vi "parse_GPGSA.vi"(0 "NMEA GPGSA String":string) -> (1 "2D3D_Automatic?":bool, 2 "New Fix Quality":T1, 3 "Valid GPS Fix?":bool)   [LabVIEW 2010]
doc: "Pass this VI an NMEA sentence and it will parse it as if it's a GPGGA sentence.\nThe Valid GPS output will be false if there's no fix or if it's not a GPGGA sentence."
uses:
  _types/FixQuality.ctl
panel:
  out "$GPGGA Code":string
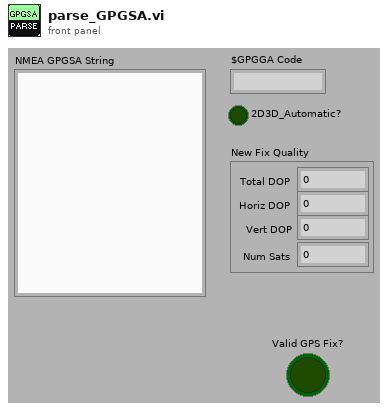
[diagram p1: front panel]
types:
  T1 = typedef "FixQuality.ctl" = cluster{"Horiz DOP":dbl, "Vert DOP":dbl, "Total DOP":dbl, "Num Sats":i32}
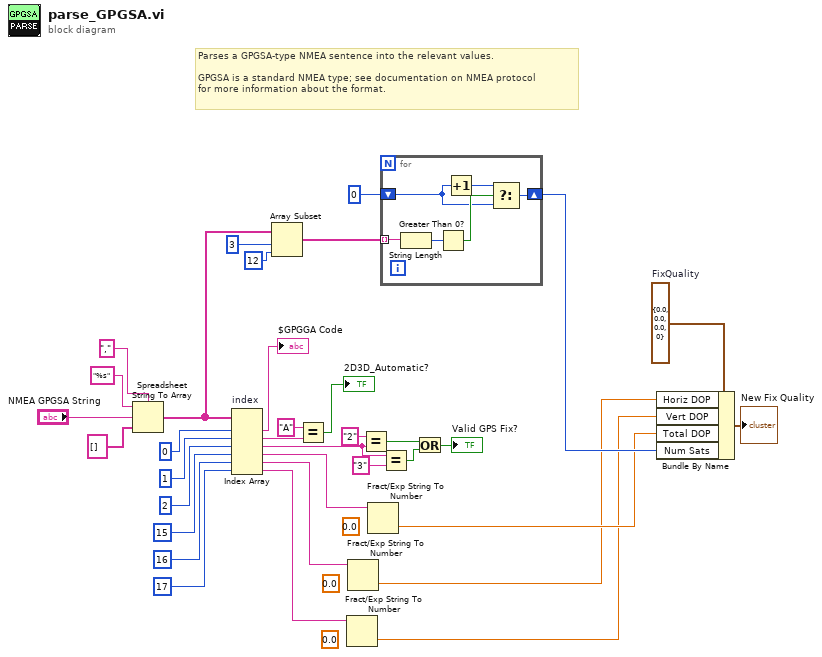
[diagram p0: block diagram]
diagram:
  (unwired) 0.0
  (unwired) 0.0
  w8 = T1 {"Horiz DOP"=0.0, "Vert DOP"=0.0, "Total DOP"=0.0, "Num Sats"=0}  # FixQuality
  (unwired) 0.0
  # "Parses a GPGSA-type NMEA sentence into the relevant values.\n\nGPGSA is a standard NMEA type; see documentation on NMEA protocol\nfor more information about the format."
  n1 = Spreadsheet String To Array(delimiter (Tab)=",", format string="%s", spreadsheet string="NMEA GPGSA String", array type (2D Dbl)=string[] []) -> (array=w13:string[])
  n2 = Index Array "index"(array=w13, index #1=0 ("index"), index #2=1 ("index"), index #3=2 ("index"), index #4=15 ("index"), index #5=16 ("index"), index #6=17 ("index")) -> (element #1=→"$GPGGA Code":string, element #2=w22:string, element #3=w18:string, element #4=w6:string, element #5=w4:string, element #6=w3:string)
  n3 = Array Subset(array=w13, index=3, length=12) -> (w10:string[])
  n4 = Equal?(x="A", y=w22) -> (x = y?=→"2D3D_Automatic?":bool)
  n5 = Fract/Exp String To Number(string=w3) -> (number=w2:dbl)  [unwired: 3 in, 1 out]
  n6 = Fract/Exp String To Number(string=w4) -> (number=w5:dbl)  [unwired: 3 in, 1 out]
  n7 = Equal?(x="2", y=w18) -> (x = y?=w16:bool)
  n8 = Fract/Exp String To Number(string=w6) -> (number=w33:dbl)  [unwired: 3 in, 1 out]
  n9 = for {
    tunnel: w10 -> [w40] mode=indexing
    shift-right: [w35] -> w34
    shift-left: 0 -> [w36]
    n10 = String Length(string=w40) -> (length=w39:i32)
    n11 = Greater Than 0?(x=w39) -> (x > 0?=w38:bool)
    n12 = Increment(x=w36) -> (x+1=w37:i32)
    n13 = Select(t=w37, s=w38, f=w36) -> (s? t:f=w35:i32)
  }
  n14 = Equal?(x=w18, y="3") -> (x = y?=w15:bool)
  n15 = Or(x=w16, y=w15) -> (x .or. y?=→"Valid GPS Fix?":bool)
  n16 = Bundle By Name(cluster=w8, "Horiz DOP"=w5, "Vert DOP"=w2, "Total DOP"=w33, "Num Sats"=w34) -> (→"New Fix Quality":T1)
